vi "status_window.vi"() -> ()   [LabVIEW 2018]
doc: "message window"
uses:
  global variables.vi
  Classes/PrepLineObject/PrepLineObject.lvclass
panel:
  in  "clear all button":bool
  in  "clear this button":bool
  in  "plot selector":string(combo)
  out "XY Graph":cluster{"X":dbl, "Y":dbl}[](graph)
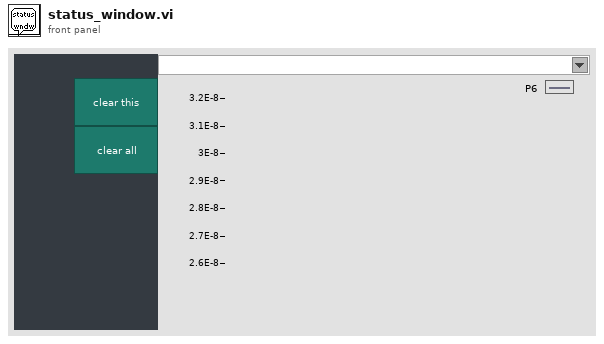
[diagram p1: front panel]
types:
  T1 = typedef "LVRectTypeDef.ctl" = cluster{"Left":i16, "Top":i16, "Right":i16, "Bottom":i16}
  T2 = cluster{"left":dbl, "top":dbl, "right":dbl, "bott":dbl}
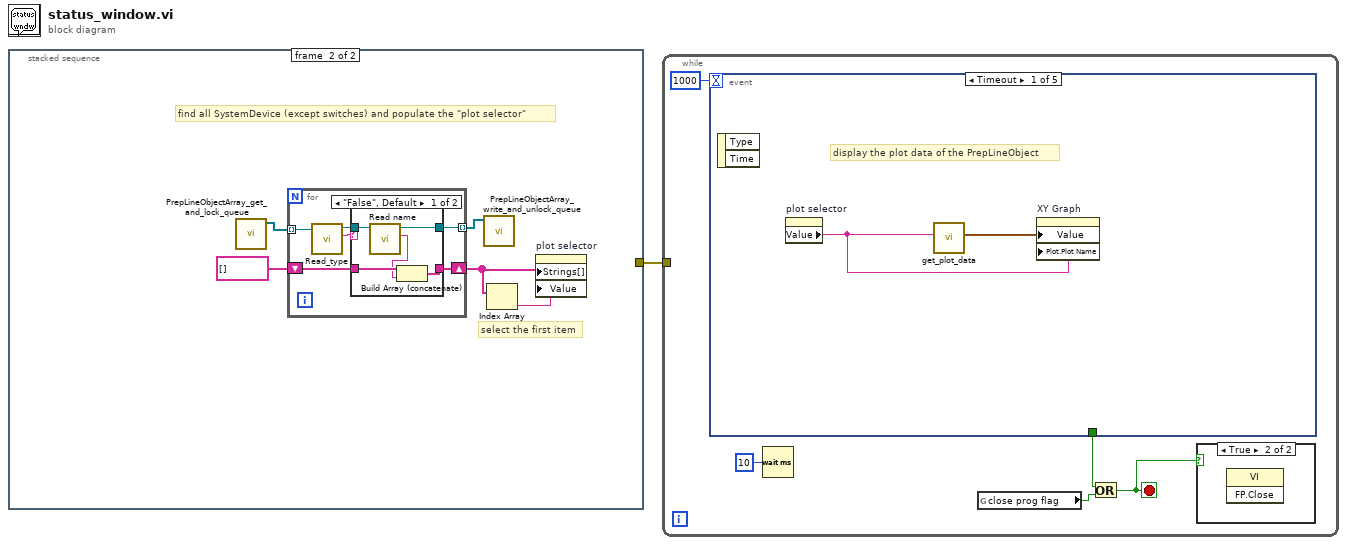
[diagram p0: block diagram]
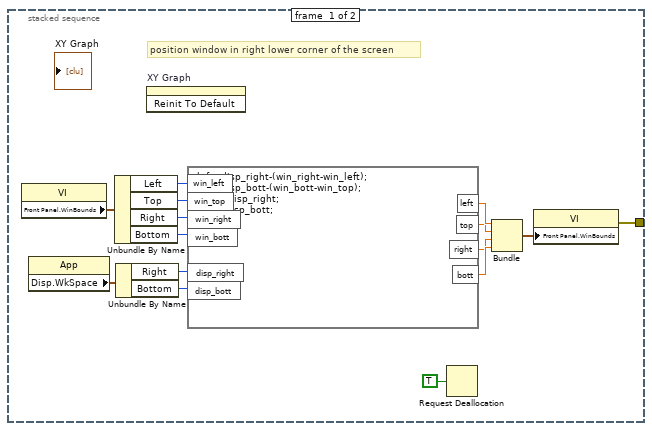
[diagram p2: hidden frame]
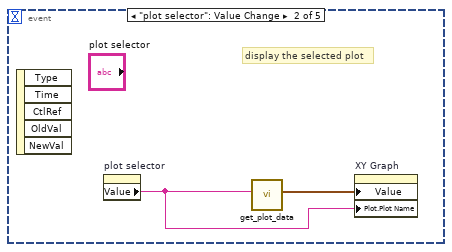
[diagram p5: hidden frame]
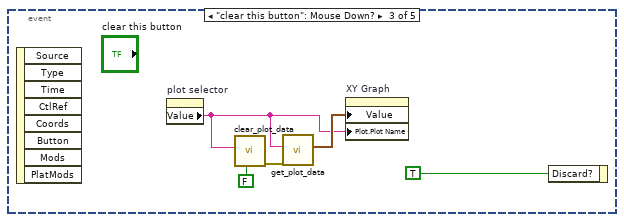
[diagram p6: hidden frame]
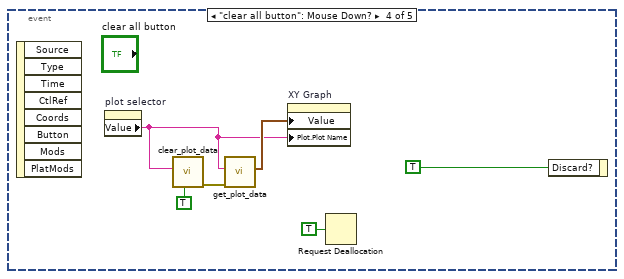
[diagram p7: hidden frame]
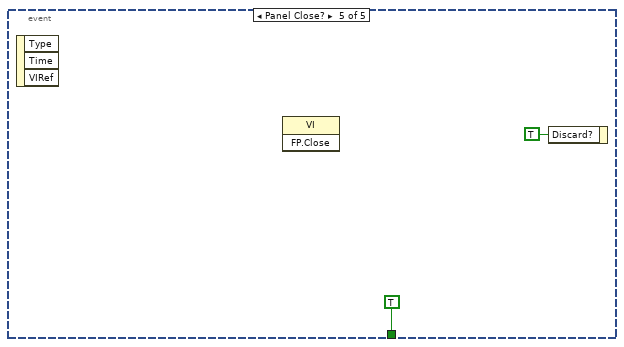
[diagram p8: hidden frame]
diagram:
  n1 = stacked-sequence {
    tunnel: [w16 _] -> w1
    frame #0 {
      # "position window in right lower corner of the screen"
      n2 = property class="VI"() -> ("Front Panel.WinBounds"=w15:T1)  [unwired: 2 in, 2 out]
      n3 = property class="App"() -> ("Disp.WkSpace"=w14:T1)  [unwired: 2 in, 2 out]
      n4 = Unbundle By Name(w15) -> ("Left"=w12:i16, "Top"=w11:i16, "Right"=w10:i16, "Bottom"=w9:i16)
      n5 = Unbundle By Name(w14) -> ("Right"=w8:i16, "Bottom"=w7:i16)
      n6 = invoke on="XY Graph" class="XYGraph (strict)" method="Reinit To Default"() -> ()  [unwired: 3 in, 3 out]
      n7 = formula code="left=disp_right-(win_right-win_left);\ntop=disp_bott-(win_bott-win_top);\nright=disp_right;\nbott=disp_bott;"("win_left"=w12, "win_top"=w11, "win_right"=w10, "win_bott"=w9, "disp_right"=w8, "disp_bott"=w7) -> ("left"=w6:dbl, "top"=w4:dbl, "right"=w3:dbl, "bott"=w5:dbl)
      n8 = Request Deallocation(TRUE ("flag")) -> ()
      n9 = Bundle("left"=w6, "top"=w4, "right"=w3, "bott"=w5) -> (w13:T2)  [unwired: 1 in]
      n10 = property class="VI"("Front Panel.WinBounds"=w13) -> (error out=w16:errorcluster)  [unwired: 2 in, 1 out]
    }
    frame #1 {
      # "select the first item"
      # "find all SystemDevice (except switches) and populate the \"plot selector\""
      n11 = call "PrepLineObjectArray_get_and_lock_queue.vi"() -> ("PrepLineObjects"=w18:refnum<class "PrepLineObject.lvclass">[])  [unwired: 10 in, 1 out]
      n12 = for {
        tunnel: w18 -> [w27] mode=indexing
        shift-right: [w23] -> w20
        shift-left: string[] [] -> [w24]
        tunnel: [w22] -> w17 mode=indexing
        n13 = call-dynamic "Read_type.vi"("PrepLinePictureObjects in"=w27) -> ("type"=w26:string, "PrepLinePictureObjects out"=w25:refnum<class "PrepLineObject.lvclass">)  [unwired: 8 in, 1 out]
        n14 = case shown="\"False\", Default" w26 {
          tunnel: w25 -> [w32 w33]
          tunnel: w24 -> [w31 w34]
          tunnel: [w30 w34] -> w23
          tunnel: [w28 w33] -> w22
          frame "False", Default {
            n15 = call-dynamic "Read name.vi"("PrepLineObject in"=w32) -> ("name"=w29:string, "PrepLineObject out"=w28:refnum<class "PrepLineObject.lvclass">)  [unwired: 8 in, 1 out]
            n16 = Build Array (concatenate)(w31, w29) -> (w30:string[])
          }
          frame "switch" {
          }
        }
      }
      n17 = call "PrepLineObjectArray_write_and_unlock_queue.vi"("PrepLineObjArray"=w17) -> ()  [unwired: 10 in, 1 out]
      n18 = Index Array(array=w20) -> (element=w19:string)  [unwired: 1 in]
      n19 = property on="plot selector" class="CmbBox"("Strings[]"=w20, "Value"=w19) -> ()  [unwired: 2 in, 2 out]
    }
  }
  n20 = while {
    tunnel: w1 -> [_]
    stop <- w35 stop-if-true
    n21 = event shown="[0] Timeout" {
      selector: _ -> [_ _ _ _ _]
      dyn-events: _ -> [_ _ _ _ _]
      timeout: 1000 -> [_ _ _ _ _]
      tunnel: [_ _ _ _ TRUE] -> w36
      event Timeout {
        # "display the plot data of the PrepLineObject"
        n22 = event-data() -> ()  [unwired: 1 in, 2 out]
        n23 = property on="plot selector" class="CmbBox"() -> ("Value"=w40:string)  [unwired: 2 in, 2 out]
        n24 = call "get_plot_data.vi"("PrepLineObjectName"=w40) -> ("value history"=w41:cluster{"time as number":dbl, "Value":dbl}[])  [unwired: 9 in, 1 out]
        n25 = property on="XY Graph" class="XYGraph (strict)"("Value"=w41, "Plot.Plot Name"=w40) -> ()  [unwired: 2 in, 2 out]
      }
      event "plot selector": Value Change {
        # "display the selected plot"
        n26 = event-data() -> ()  [unwired: 1 in, 5 out]
        n27 = property on="plot selector" class="CmbBox"() -> ("Value"=w42:string)  [unwired: 2 in, 2 out]
        n28 = call "get_plot_data.vi"("PrepLineObjectName"=w42) -> ("value history"=w43:cluster{"time as number":dbl, "Value":dbl}[])  [unwired: 9 in, 1 out]
        n29 = property on="XY Graph" class="XYGraph (strict)"("Value"=w43, "Plot.Plot Name"=w42) -> ()  [unwired: 2 in, 2 out]
      }
      event "clear this button": Mouse Down? {
        n30 = event-data() -> ()  [unwired: 1 in, 8 out]
        n31 = property on="plot selector" class="CmbBox"() -> ("Value"=w44:string)  [unwired: 2 in, 2 out]
        n32 = call "clear_plot_data.vi"("clear all?"=FALSE, "PrepLineObjectName"=w44) -> ("error out"=w45:errorcluster)  [unwired: 9 in]
        n33 = call "get_plot_data.vi"("error in (no error)"=w45, "PrepLineObjectName"=w44) -> ("value history"=w46:cluster{"time as number":dbl, "Value":dbl}[])  [unwired: 8 in, 1 out]
        n34 = property on="XY Graph" class="XYGraph (strict)"("Value"=w46, "Plot.Plot Name"=w44) -> ()  [unwired: 2 in, 2 out]
        n35 = event-data("Discard?"=TRUE) -> ()  [unwired: 1 in, 1 out]
      }
      event "clear all button": Mouse Down? {
        n36 = event-data() -> ()  [unwired: 1 in, 8 out]
        n37 = property on="plot selector" class="CmbBox"() -> ("Value"=w50:string)  [unwired: 2 in, 2 out]
        n38 = call "clear_plot_data.vi"("clear all?"=TRUE, "PrepLineObjectName"=w50) -> ("error out"=w51:errorcluster)  [unwired: 9 in]
        n39 = call "get_plot_data.vi"("error in (no error)"=w51, "PrepLineObjectName"=w50) -> ("value history"=w52:cluster{"time as number":dbl, "Value":dbl}[])  [unwired: 8 in, 1 out]
        n40 = property on="XY Graph" class="XYGraph (strict)"("Value"=w52, "Plot.Plot Name"=w50) -> ()  [unwired: 2 in, 2 out]
        n41 = Request Deallocation(TRUE ("flag")) -> ()
        n42 = event-data("Discard?"=TRUE) -> ()  [unwired: 1 in, 1 out]
      }
      event Panel Close? {
        n43 = event-data() -> ()  [unwired: 1 in, 3 out]
        n44 = invoke class="VI" method="FP.Close"() -> ()  [unwired: 3 in, 3 out]
        n45 = event-data("Discard?"=TRUE) -> ()  [unwired: 1 in, 1 out]
      }
    }
    n46 = Wait (ms)(milliseconds to wait=u32 10) -> ()  [unwired: 1 out]
    n47 = global read "global variables.vi" "close prog flag"() -> (w37:bool)
    n48 = Or(x=w36, y=w37) -> (x .or. y?=w35:bool)
    n49 = case shown="True" w35 {
      frame False {
      }
      frame True {
        n50 = invoke class="VI" method="FP.Close"() -> ()  [unwired: 3 in, 3 out]
      }
    }
  }
